vi "ReadLabVIEWVNA.vi"() -> ()   [LabVIEW 2020]
panel:
  out "output cluster":T1
  out "string array 2":string[][](array[string])
  out "string array":string[](array[string])
  out "after substring":string
  out "text":string
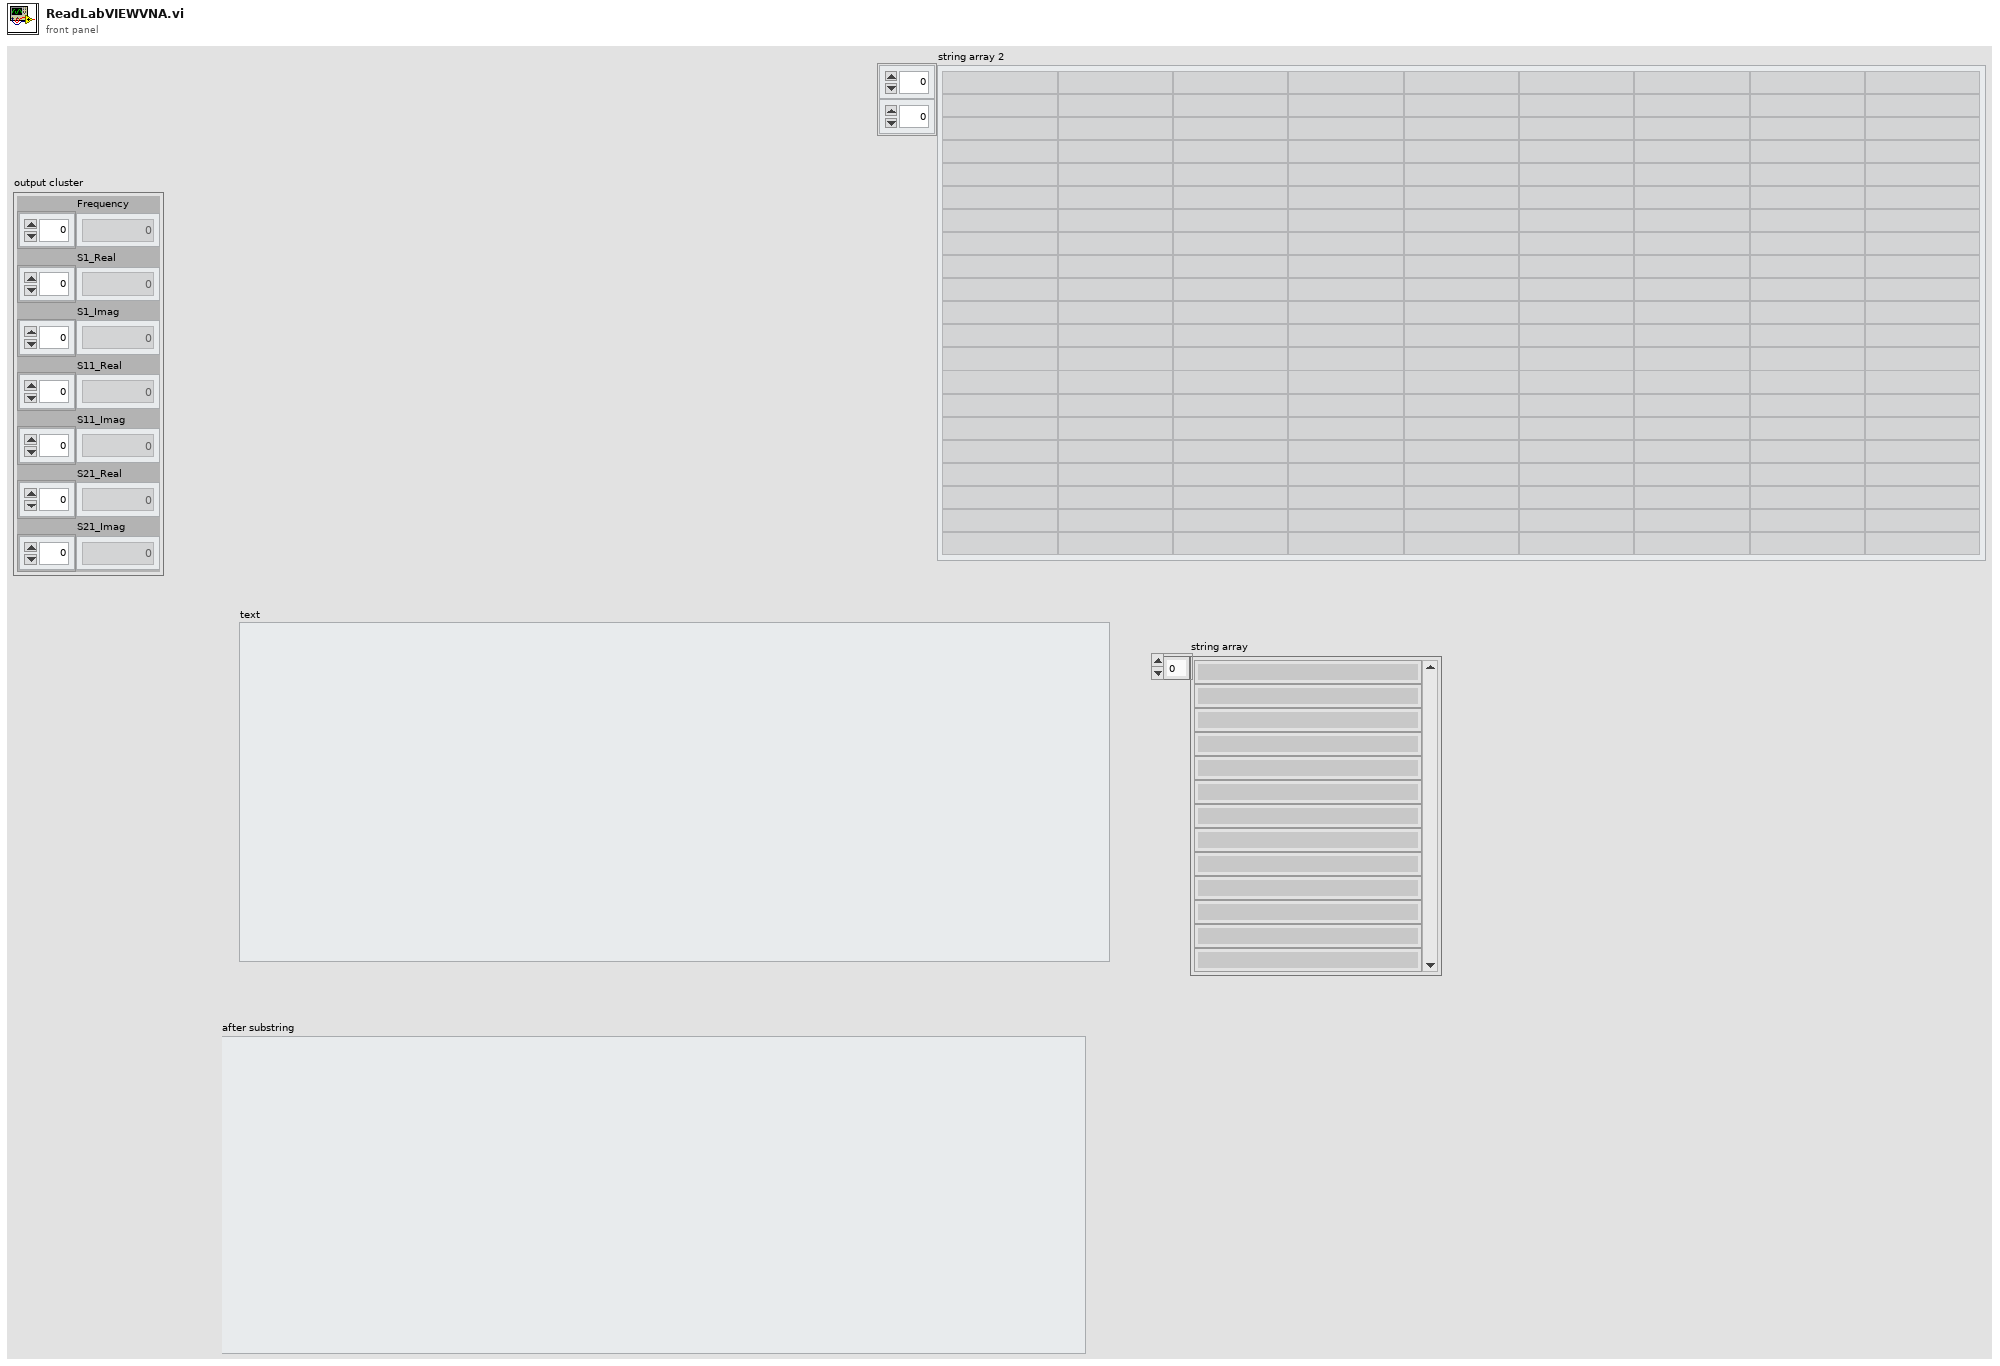
[diagram p1: front panel]
types:
  T1 = cluster{"Frequency":dbl[], "S1_Real":dbl[], "S1_Imag":dbl[], "S11_Real":dbl[], "S11_Imag":dbl[], "S21_Real":dbl[], "S21_Imag":dbl[]}
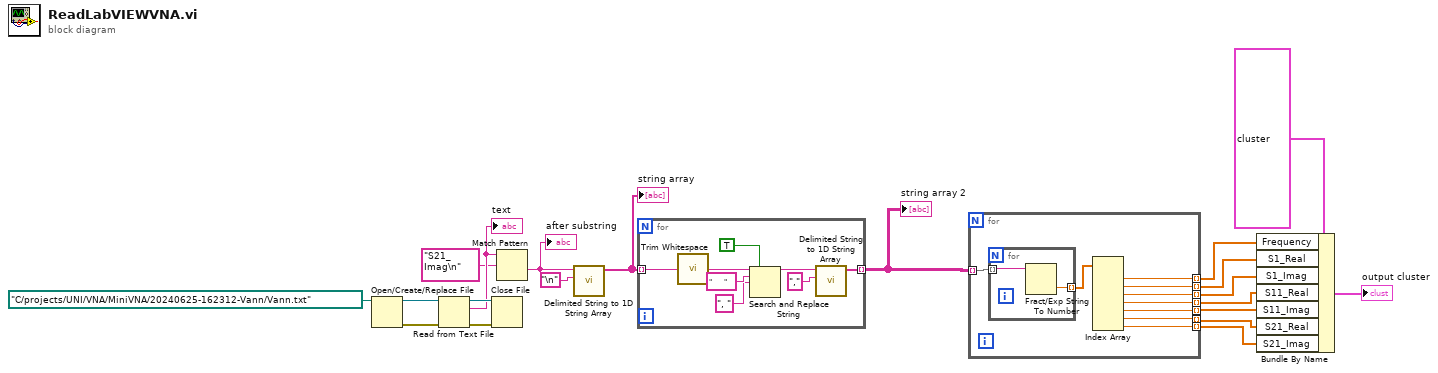
[diagram p0: block diagram]
diagram:
  n1 = Open/Create/Replace File(file path (use dialog)=path "C:/projects/UNI/VNA/MiniVNA/20240625-162312-Vann/Vann.txt" ("file path (dialog if empty)")) -> (refnum out=w20:refnum<file>, error out=w17:errorcluster)  [unwired: 5 in, 1 out]
  n2 = Read from Text File(file (use dialog)=w20, error in=w17) -> (refnum out=w19:refnum<file>, text=w15:string, error out=w18:errorcluster)  [unwired: 2 in, 1 out]
  "text" <- w15
  n3 = Close File(refnum=w19, error in=w18) -> ()  [unwired: 2 out]
  n4 = Match Pattern(string=w15, regular expression="S21_Imag\n" ("search string/char (-)")) -> (after substring=w11:string)  [unwired: 1 in, 3 out]
  "after substring" <- w11
  n5 = call <vilib>:"Delimited String to 1D String Array.vi"("delimiter"="\n", "delimited string"=w11) -> ("string array"=w12:string[])  [unwired: 9 in]
  "string array" <- w12
  n6 = for {
    tunnel: w12 -> [w28] mode=indexing
    tunnel: [w27] -> w10 mode=indexing
    n7 = call <vilib>:"Trim Whitespace.vi"("string"=w28) -> ("trimmed string"=w26:string)  [unwired: 1 in]
    n8 = Search and Replace String(replace all?=TRUE ("replace all? (F)"), input string=w26, search string="      ", replace string=", " ("replace string (\"\")")) -> (result string=w21:string)  [unwired: 4 in, 3 out]
    n9 = call <vilib>:"Delimited String to 1D String Array.vi"("delimiter"=",", "delimited string"=w21) -> ("string array"=w27:string[])  [unwired: 9 in]
  }
  "string array 2" <- w10
  n10 = for {
    tunnel: w10 -> [w37] mode=indexing
    tunnel: [w35] -> w9 mode=indexing
    tunnel: [w34] -> w8 mode=indexing
    tunnel: [w33] -> w7 mode=indexing
    tunnel: [w32] -> w6 mode=indexing
    tunnel: [w31] -> w5 mode=indexing
    tunnel: [w30] -> w4 mode=indexing
    tunnel: [w29] -> w3 mode=indexing
    n11 = for {
      tunnel: w37 -> [w39] mode=indexing
      tunnel: [w38] -> w36 mode=indexing
      n12 = Fract/Exp String To Number(string=w39) -> (number=w38:dbl)  [unwired: 3 in, 1 out]
    }
    n13 = Index Array(array=w36) -> (element #1=w35:dbl, element #2=w34:dbl, element #3=w33:dbl, element #4=w32:dbl, element #5=w31:dbl, element #6=w30:dbl, element #7=w29:dbl)  [unwired: 7 in]
  }
  n14 = Bundle By Name(cluster=T1 {"Frequency"=array[802 elements], "S1_Real"=array[802 elements], "S1_Imag"=array[802 elements], "S11_Real"=array[802 elements], "S11_Imag"=array[802 elements], "S21_Real"=array[802 elements], "S21_Imag"=array[802 elements]} ("output cluster"), "Frequency"=w9, "S1_Real"=w8, "S1_Imag"=w7, "S11_Real"=w6, "S11_Imag"=w5, "S21_Real"=w4, "S21_Imag"=w3) -> (→"output cluster":T1)
